vi "Queue State Machine.vi"   [LabVIEW 2020]
uses:
  SubVI/Queue Create.vi
  SubVI/Queue Remove.vi
  SubVI/Queue Destroy.vi
panel:
  # "队列\n状态机"
types:
  T1 = cluster{"Error":errorcluster, "Exit":bool, "queue":string, "data":variant}
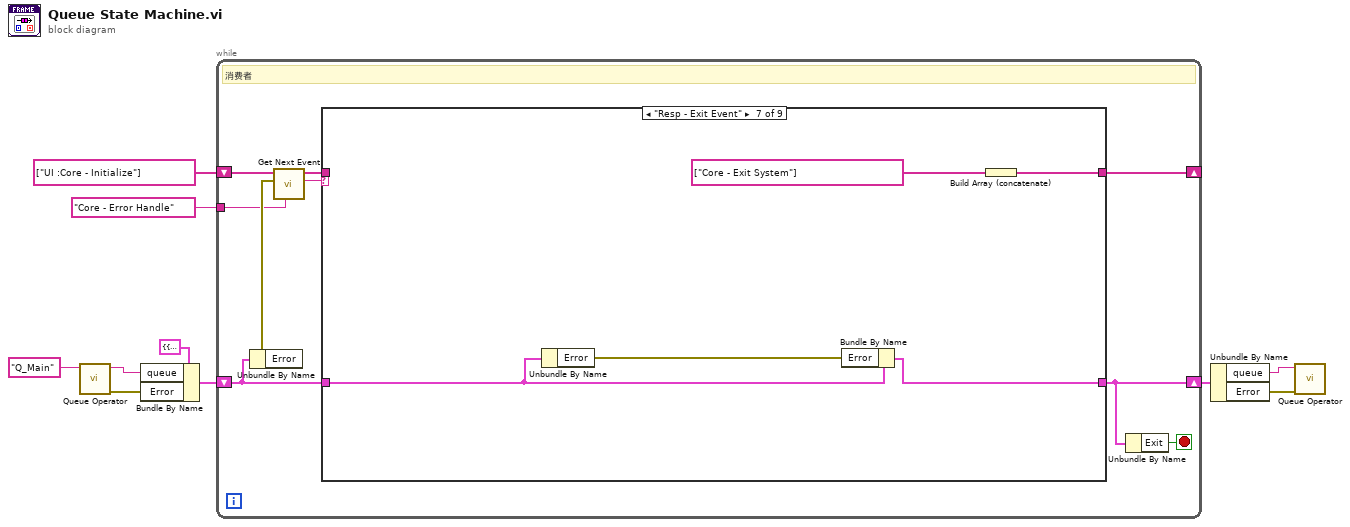
[diagram p0: block diagram]
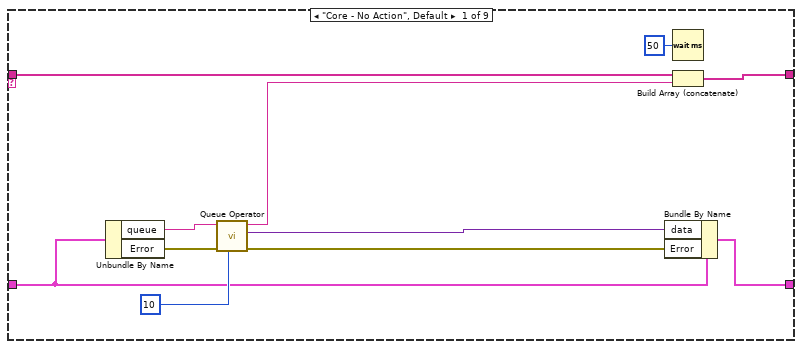
[diagram p2: hidden frame]
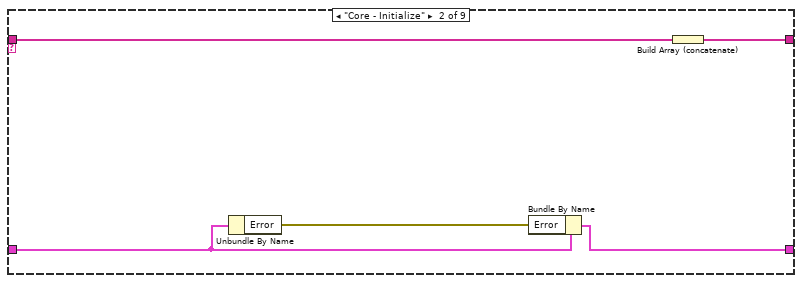
[diagram p3: hidden frame]
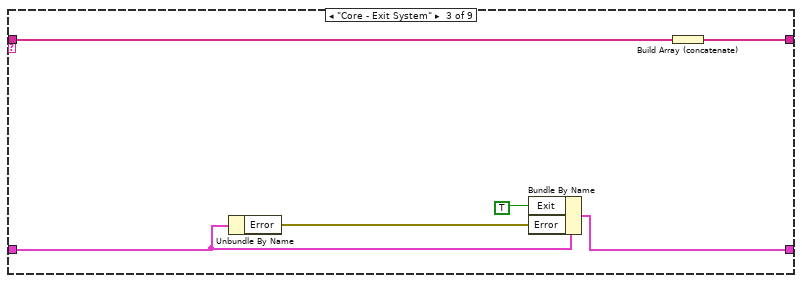
[diagram p4: hidden frame]
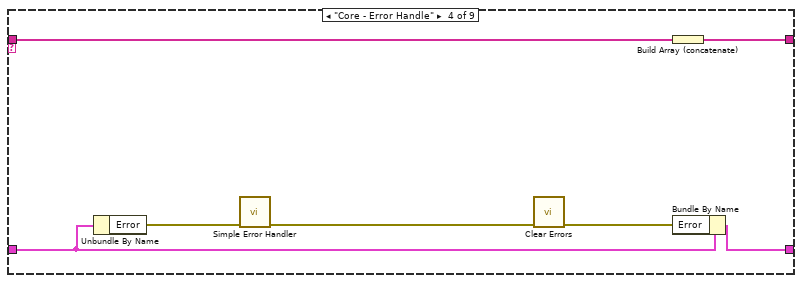
[diagram p5: hidden frame]
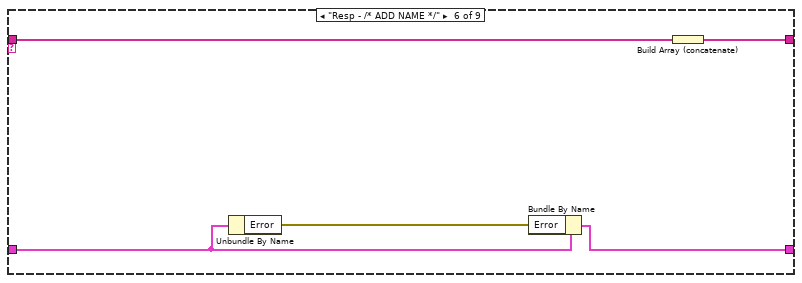
[diagram p7: hidden frame]
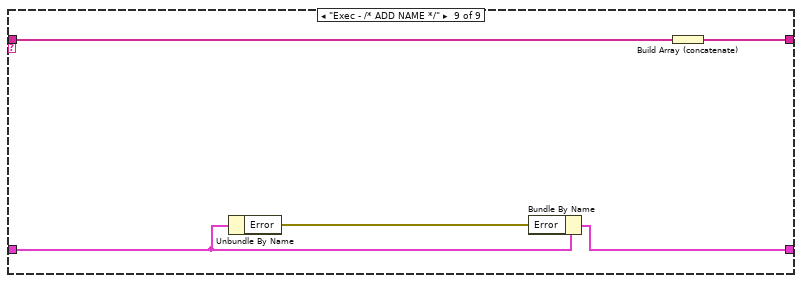
[diagram p9: hidden frame]
diagram:
  n1 = call-poly "Queue Operator.vi"("queue name in"="Q_Main") -> ("error out"=w3:errorcluster, "queue name out"=w2:string)  [unwired: 7 in, 2 out]
  n2 = Bundle By Name(cluster=T1 {"Error"={"status"=FALSE, "code"=0, "source"=""}, "Exit"=FALSE, "queue"="", "data"=variant} ("Temp Variable"), "queue"=w2, "Error"=w3) -> (w8:T1)
  n3 = while {
    shift-right: [w14] -> _
    shift-left: string[] ["UI :Core - Initialize"] -> [w17]
    shift-right: [w13] -> w6
    shift-left: w8 -> [w16]
    tunnel: "Core - Error Handle" ("Error Handle") -> [w11]
    stop <- w12 stop-if-true
    # "消费者"
    n4 = Unbundle By Name(w16) -> ("Error"=w15:errorcluster)
    n5 = call "Get Next Event.vi"("Error Handle"=w11, "error in (no error)"=w15, "event queue in"=w17) -> ("next event"=w18:string, "event queue out"=w19:string[])  [unwired: 7 in]
    n6 = case shown="\"Resp - Exit Event\"" w18 {
      tunnel: w19 -> [w27 w35 w41 w48 w50 w55 _ w62 w67]
      tunnel: w16 -> [w25 w33 w39 w46 w49 w53 w59 w61 w65]
      tunnel: [w26 w34 w40 w47 w50 w54 w60 w62 w66] -> w14
      tunnel: [w23 w31 w38 w45 w49 w52 w58 w61 w64] -> w13
      frame "Core - No Action", Default {
        n7 = Unbundle By Name(w25) -> ("queue"=w29:string, "Error"=w30:errorcluster)
        n8 = call-poly "Queue Operator.vi"("timeout(ms: -1)"=10, "error in (no error)"=w30, "queue name"=w29) -> ("error out"=w24:errorcluster, "data"=w21:variant, "event"=w22:string)  [unwired: 5 in, 1 out]
        n9 = Bundle By Name(cluster=w25, "data"=w21, "Error"=w24) -> (w23:T1)
        n10 = Wait (ms)(milliseconds to wait=u32 50 ("等待时间（毫秒）")) -> ()  [unwired: 1 out]
        n11 = Build Array (concatenate)(w27, w22) -> (w26:string[])
      }
      frame "Core - Initialize" {
        n12 = Unbundle By Name(w33) -> ("Error"=w32:errorcluster)
        n13 = Bundle By Name(cluster=w33, "Error"=w32) -> (w31:T1)
        n14 = Build Array (concatenate)(w35) -> (w34:string[])
      }
      frame "Core - Exit System" {
        n15 = Unbundle By Name(w39) -> ("Error"=w37:errorcluster)
        n16 = Bundle By Name(cluster=w39, "Exit"=TRUE, "Error"=w37) -> (w38:T1)
        n17 = Build Array (concatenate)(w41) -> (w40:string[])
      }
      frame "Core - Error Handle" {
        n18 = Unbundle By Name(w46) -> ("Error"=w43:errorcluster)
        n19 = call <vilib>:"Simple Error Handler.vi"("error in (no error)"=w43) -> ("error out"=w42:errorcluster)  [unwired: 4 in, 4 out]
        n20 = call <vilib>:"Clear Errors.vi"("error in (no error)"=w42) -> ("error out"=w44:errorcluster)  [unwired: 5 in, 1 out]
        n21 = Build Array (concatenate)(w48) -> (w47:string[])
        n22 = Bundle By Name(cluster=w46, "Error"=w44) -> (w45:T1)
      }
      frame "---------------------------------Response---------------------------------" {
      }
      frame "Resp - /* ADD NAME */" {
        n23 = Unbundle By Name(w53) -> ("Error"=w51:errorcluster)
        n24 = Bundle By Name(cluster=w53, "Error"=w51) -> (w52:T1)
        n25 = Build Array (concatenate)(w55) -> (w54:string[])
      }
      frame "Resp - Exit Event" {
        n26 = Unbundle By Name(w59) -> ("Error"=w57:errorcluster)
        n27 = Bundle By Name(cluster=w59, "Error"=w57) -> (w58:T1)
        n28 = Build Array (concatenate)(string[] ["Core - Exit System"]) -> (w60:string[])
      }
      frame "----------------------------------Execute-----------------------------------" {
      }
      frame "Exec - /* ADD NAME */" {
        n29 = Unbundle By Name(w65) -> ("Error"=w63:errorcluster)
        n30 = Bundle By Name(cluster=w65, "Error"=w63) -> (w64:T1)
        n31 = Build Array (concatenate)(w67) -> (w66:string[])
      }
    }
    n32 = Unbundle By Name(w13) -> ("Exit"=w12:bool)
  }
  n33 = Unbundle By Name(w6) -> ("queue"=w4:string, "Error"=w5:errorcluster)
  n34 = call-poly "Queue Operator.vi"("error in (no error)"=w5, "queue name in"=w4) -> ()  [unwired: 8 in, 2 out]
